vi "Change Unit.vi"(0 "Waveforms Common Methods in":refnum<class "Waveforms Common Methods.lvclass">, 9 "ParamTags":T1, 11 "error in (no error)":errorcluster, 12 "New Value":u16, 14 "Old Value":u16) -> (4 "Waveforms Common Methods out":refnum<class "Waveforms Common Methods.lvclass">, 15 "error out":errorcluster)   [LabVIEW 2021, in "Rigol DG822 UI.lvlib" / "Waveforms Common Methods.lvclass"]
uses:
  Waveforms Common Methods.lvclass
  lib/controls.llb/WaveformParamTags.ctl
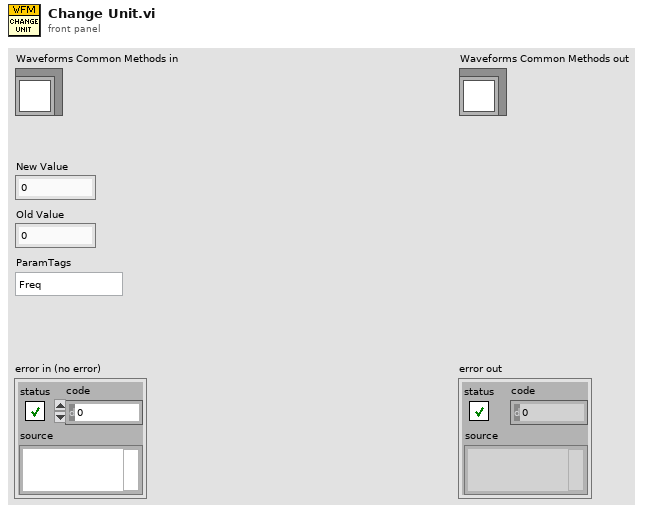
[diagram p1: front panel]
types:
  T1 = typedef "WaveformParamTags.ctl" = enum16{"Freq", "Period", "Ampl", "HighL", "Offset", "LowL", "Phase", "Duty", "Width", "RisEdge", "FallEdge"}
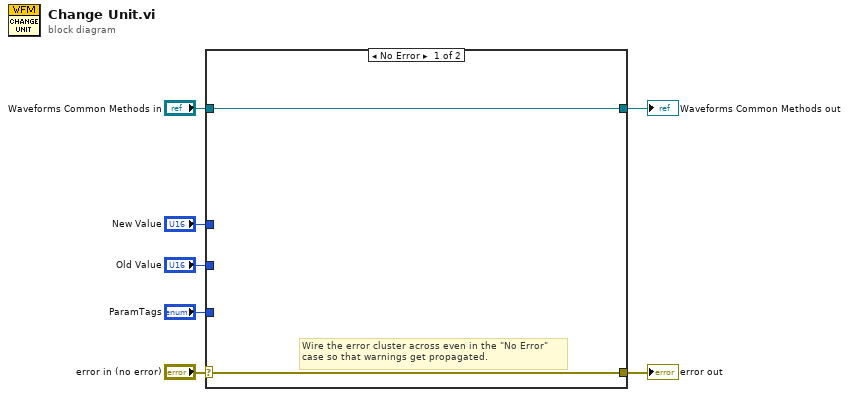
[diagram p0: block diagram]
diagram:
  n1 = case shown="No Error" "error in (no error)" {
    selector: "error in (no error)" -> [w8 w11]
    tunnel: [w8 w11] -> w6
    tunnel: [w9 w10] -> w4
    tunnel: "Waveforms Common Methods in" -> [w9 w10]
    tunnel: "ParamTags" -> [_ _]
    tunnel: "New Value" -> [_ _]
    tunnel: "Old Value" -> [_ _]
    frame No Error {
      # "Wire the error cluster across even in the \"No Error\"\ncase so that warnings get propagated."
    }
    frame Error {
    }
  }
  "error out" <- w6
  "Waveforms Common Methods out" <- w4
